vi "configDigitalOutput.vi"(8 "error in (no error)":errorcluster, 9 "Physical Channels":string, 10 "name":string="0", 11 "DigitalOutput in":refnum<class "DigitalOutput.lvclass">) -> (0 "error out":errorcluster, 3 "DigitalOutput out":refnum<class "DigitalOutput.lvclass">)   [LabVIEW 2011, in "Hardware.lvlib" / "Channels.lvlib" / "DigitalOutput.lvclass"]
doc: "Use this vi to set the name, and physical channels needed for the digital output. This vi then communicates with the actual device (via its child objects, DIO64Output etc) to set these properties."
uses:
  DigitalOutput.lvclass
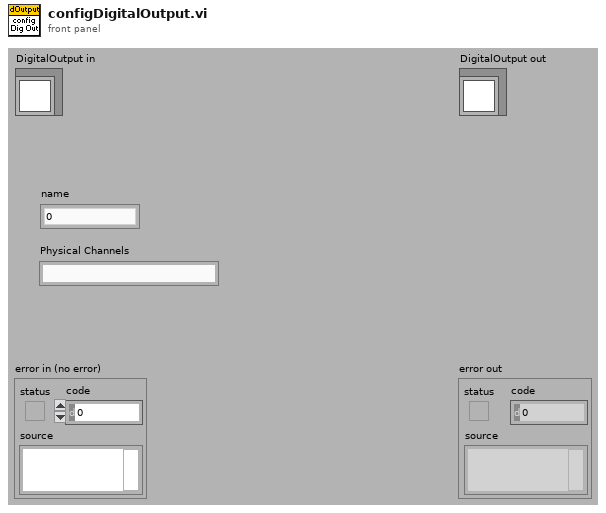
[diagram p1: front panel]
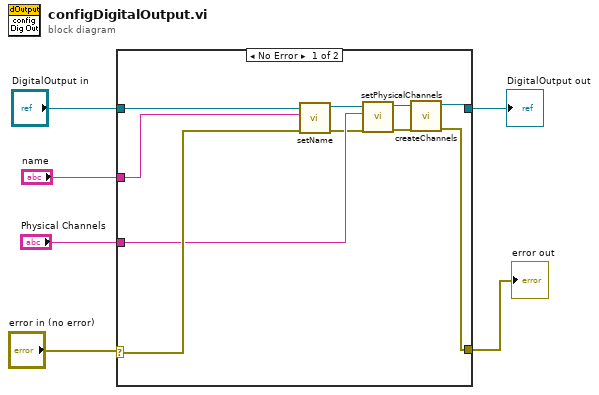
[diagram p0: block diagram]
diagram:
  n1 = case shown="No Error" "error in (no error)" {
    selector: "error in (no error)" -> [w15 w18]
    tunnel: [w13 w18] -> w5
    tunnel: [w14 w17] -> w3
    tunnel: "DigitalOutput in" -> [w16 w17]
    tunnel: "name" -> [w7 _]
    tunnel: "Physical Channels" -> [w11 _]
    frame No Error {
      n2 = call-dynamic "setName.vi"("error in (no error)"=w15, "name"=w7, "DigitalOutput.lvclass in"=w16) -> ("error out"=w10:errorcluster, "DigitalOutput.lvclass out"=w12:refnum<class "DigitalOutput.lvclass">)  [unwired: 7 in]
      n3 = call-dynamic "setPhysicalChannels.vi"("error in (no error)"=w10, "Physical Channels"=w11, "DigitalOutput.lvclass in"=w12) -> ("error out"=w8:errorcluster, "DigitalOutput.lvclass out"=w9:refnum<class "DigitalOutput.lvclass">)  [unwired: 7 in]
      n4 = call-dynamic "createChannels.vi"("error in (no error)"=w8, "DigitalOutput in"=w9) -> ("error out"=w13:errorcluster, "DigitalOutput out"=w14:refnum<class "DigitalOutput.lvclass">)  [unwired: 8 in]
    }
    frame Error {
    }
  }
  "error out" <- w5
  "DigitalOutput out" <- w3
